vi "Toggle Relay.vi"(4 "Simulate":bool, 6 "timeout":dbl=10.0 format="%0.2f", 8 "error in":errorcluster, 9 "InitialState (T)":bool=TRUE, 10 "ToggleWaitIntv (250ms)":u32=250, 11 "DO-Line Ref":refnum<k21>) -> (0 "error out":errorcluster, 3 "DO-Line Ref out":refnum<k21>)   [LabVIEW 2022 SP3, in "DAQ.lvclass"]
doc: "Developed by Kevin Thompson\nkevin@thompsonengineering.net\n\nCopyright 2018-2020\nThompson Engineering, LLC"
uses:
  DAQ.lvclass
  DAQ.lvclass/DAQ.ctl
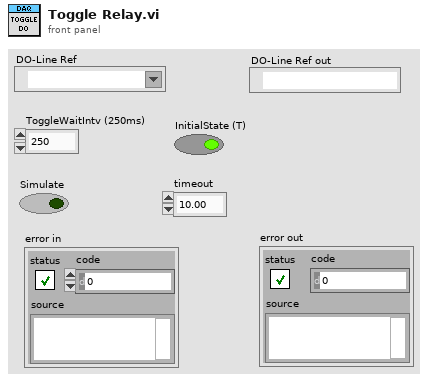
[diagram p1: front panel]
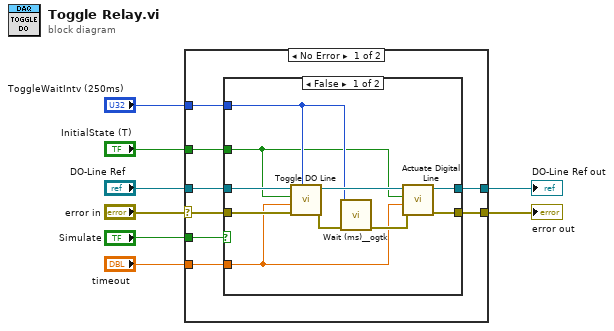
[diagram p0: block diagram]
diagram:
  n1 = case shown="No Error" "error in" {
    selector: "error in" -> [w13 w30]
    tunnel: "DO-Line Ref" -> [w16 w29]
    tunnel: "ToggleWaitIntv (250ms)" -> [w15 _]
    tunnel: [w14 w30] -> w6
    tunnel: [w12 w29] -> w4
    tunnel: "InitialState (T)" -> [w11 _]
    tunnel: "timeout" -> [w10 _]
    tunnel: "Simulate" -> [w9 _]
    frame No Error {
      n2 = case shown="False" w9 {
        tunnel: w16 -> [w24 w28]
        tunnel: w15 -> [w22 _]
        tunnel: [w21 w27] -> w14
        tunnel: w13 -> [w20 w27]
        tunnel: [w19 w28] -> w12
        tunnel: w11 -> [w18 _]
        tunnel: w10 -> [w17 _]
        frame False {
          n3 = call "Toggle DO Line.vi"("ToggleWaitIntv (ms)"=w22, "error in"=w20, "timeout"=w17, "InitialState"=w18, "DO-Line Ref"=w24) -> ("error out"=w26:errorcluster, "DO-Line Ref out"=w23:refnum<k21>)  [unwired: 5 in]
          n4 = call <userlib>:"Wait (ms)__ogtk.vi"("error in (no error)"=w26, "milliseconds to wait"=w22) -> ("error out"=w25:errorcluster)  [unwired: 8 in, 1 out]
          n5 = call "Actuate Digital Line.vi"("error in"=w25, "timeout"=w17, "state"=w18, "DO-Line Ref"=w23) -> ("error out"=w21:errorcluster, "DO-Line Ref out"=w19:refnum<k21>)  [unwired: 6 in]
        }
        frame True {
        }
      }
    }
    frame Error {
    }
  }
  "error out" <- w6
  "DO-Line Ref out" <- w4
